vi "Append unique suffix.vi"(6 "Extention":string, 7 "Suffix":string, 8 "error in (no error)":errorcluster, 10 "ovewrite ?":bool, 11 "Path":path) -> (0 "error out":errorcluster, 3 "Path out":path)   [LabVIEW 2021]
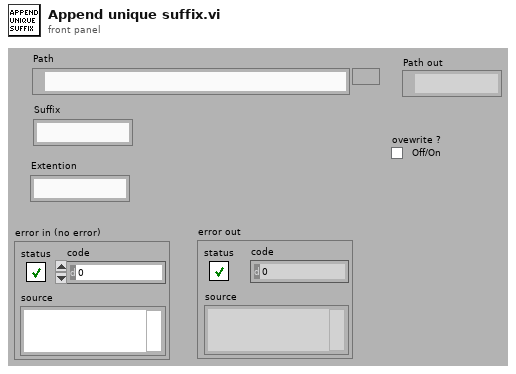
[diagram p1: front panel]
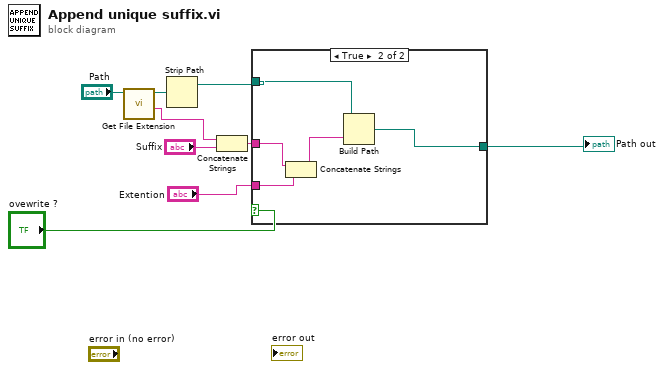
[diagram p0: block diagram]
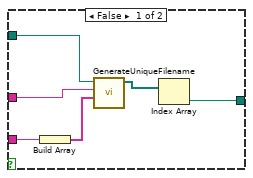
[diagram p2: hidden frame]
diagram:
  n1 = call <vilib>:"Get File Extension.vi"("file"="Path") -> ("filename without extension"=w4:string, "dup file"=w3:path)  [unwired: 6 in, 3 out]
  n2 = Strip Path(path=w3) -> (stripped path=w6:path)  [unwired: 1 out]
  n3 = Concatenate Strings(w4, "Suffix") -> (w8:string)
  n4 = case shown="True" "ovewrite ?" {
    tunnel: w8 -> [w15 w20]
    tunnel: "Extention" -> [w14 w19]
    tunnel: w6 -> [w12 w18]
    tunnel: [w10 w16] -> w2
    frame False {
      n5 = Build Array(w14) -> (w13:string[])
      n6 = call "GenerateUniqueFilename.vi"("File name suffixes"=w13, "File name prefix"=w15, "Folder Path Control"=w12) -> ("Paths"=w11:path[])  [unwired: 7 in, 1 out]
      n7 = Index Array(array=w11) -> (element=w10:path)  [unwired: 1 in]
    }
    frame True {
      n8 = Concatenate Strings(w20, w19) -> (w17:string)
      n9 = Build Path(base path=w18, name or relative path=w17) -> (appended path=w16:path)
    }
  }
  "Path out" <- w2
